vi "Call VI Reference.vi"(8 "error in":errorcluster, 11 "last level":i32=1) -> (0 "error out":errorcluster, 3 "vi reference out":refnum<vi>)   [LabVIEW 2020]
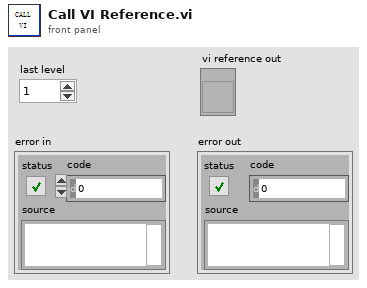
[diagram p1: front panel]
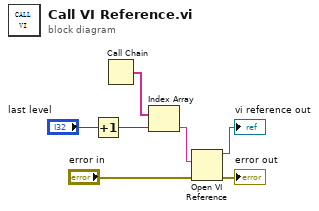
[diagram p0: block diagram]
diagram:
  n1 = Increment(x="last level") -> (x+1=w1:i32)
  n2 = Call Chain ("调用链")() -> (call chain=w4:string[])
  n3 = Index Array(array=w4, index=w1) -> (element=w2:string)
  n4 = Open VI Reference(vi path=w2, error in (no error)="error in") -> (vi reference=→"vi reference out":refnum<vi>, error out=→"error out":errorcluster)  [unwired: 4 out]
